vi "Query Edited Arbitrary Waveform.vi"(8 "error in (no error)":errorcluster, 11 "VISA resource name":refnum<visa-resource-name>) -> (0 "error out":errorcluster, 1 "Number Of Points":i32, 2 "Waveform Function":string, 3 "VISA resource name out":refnum<visa-resource-name>)   [LabVIEW 2017, in "Scope.lvlib" / "Tektronix DPO MSO 2000 4000 Series.lvlib"]
doc: "Queries the currently selected arbitrary waveform pre-defined function and the point number in the arbitrary waveform edit memory.\n\n<B>Notes:</B>\n(1) This VI is available for MDO3000 Series only.\n\n(2) Requires the MDO3AFG option to be installed."
uses:
  Tektronix DPO MSO 2000 4000 Series.lvlib
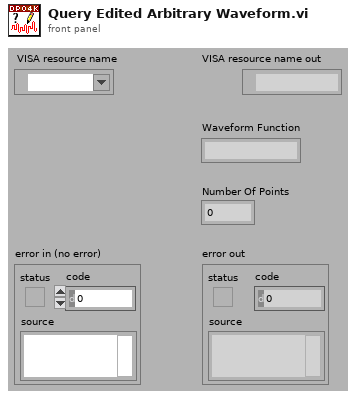
[diagram p1: front panel]
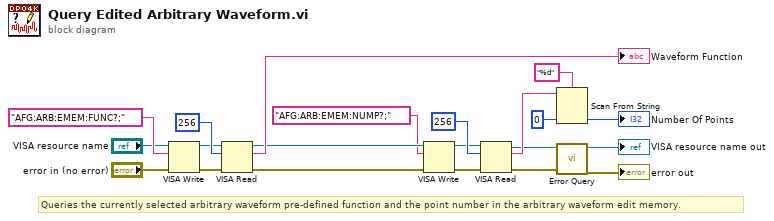
[diagram p0: block diagram]
diagram:
  # "Queries the currently selected arbitrary waveform pre-defined function and the point number in the arbitrary waveform edit memory."
  n1 = VISA Write(VISA resource name="VISA resource name", write buffer="AFG:ARB:EMEM:FUNC?;", error in (no error)="error in (no error)") -> (VISA resource name out=w12:refnum<visa-resource-name>, error out=w11:errorcluster)  [unwired: 1 out]
  n2 = VISA Read(VISA resource name=w12, byte count=u32 256, error in (no error)=w11) -> (VISA resource name out=w9:refnum<visa-resource-name>, read buffer=→"Waveform Function":string, error out=w8:errorcluster)  [unwired: 1 out]
  n3 = VISA Write(VISA resource name=w9, write buffer="AFG:ARB:EMEM:NUMP?;", error in (no error)=w8) -> (VISA resource name out=w7:refnum<visa-resource-name>, error out=w6:errorcluster)  [unwired: 1 out]
  n4 = VISA Read(VISA resource name=w7, byte count=u32 256, error in (no error)=w6) -> (VISA resource name out=w3:refnum<visa-resource-name>, read buffer=w17:string, error out=w2:errorcluster)  [unwired: 1 out]
  n5 = Scan From String(format string="%d", input string=w17, default 1=0 ("default value 1")) -> (output 1=→"Number Of Points":i32)  [unwired: 2 in, 3 out]
  n6 = call "Error Query.vi"("error in (no error)"=w2, "VISA resource name"=w3) -> ("error out"=→"error out":errorcluster, "VISA resource name out"=→"VISA resource name out":refnum<visa-resource-name>)  [unwired: 6 in, 2 out]
